vi "ep_Torque to Load.vi"(0 "air-gap torque waveform [Nm]":waveform(dbl), 1 "total input active power [W]":dbl, 5 "speed [RPM]":dbl, 11 "error in (no error)":errorcluster, 12 "initial conditions":T1) -> (3 "torque waveform [Nm]":waveform(dbl), 4 "torque [Nm]":dbl, 6 "load [W]":dbl, 8 "efficiency [%]":dbl, 14 "final conditions":T1, 15 "error out":errorcluster)   [LabVIEW 2014, in "NI_EP_Motor Monitoring.lvlib"]
uses:
  <vilib>/addons/Electrical Power/Motor Monitoring/NI_EP_Motor Monitoring.lvlib
  <vilib>/addons/Electrical Power/Motor Monitoring/subVIs/ep_Initial Conditions for Air Gap.ctl
  <vilib>/Analysis/baseanly.llb/Mean (DBL).vi
  <vilib>/Analysis/NI_AALBase.lvlib
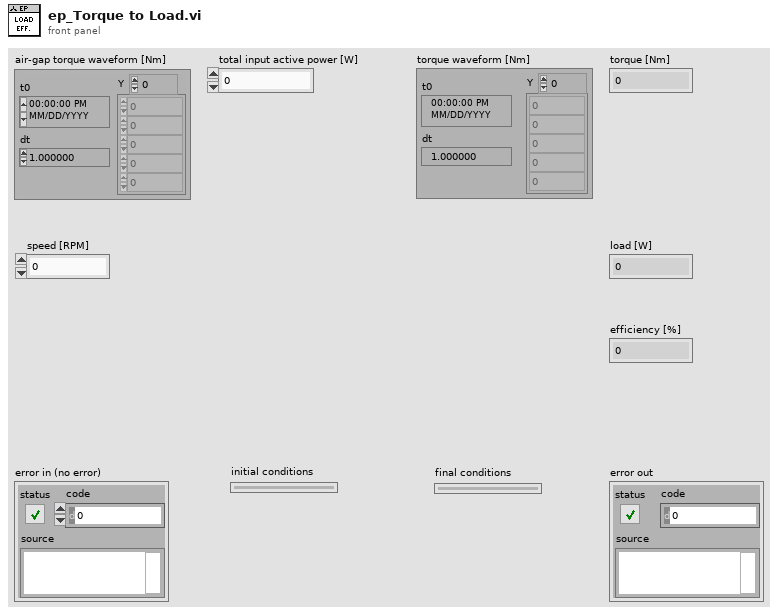
[diagram p1: front panel]
types:
  T1 = typedef "NI_EP_Motor Monitoring.lvlib/ep_Initial Conditions for Air Gap.ctl" = cluster{"integration state in A":cluster{"initial value":dbl, "initial integration":dbl}, "integration state in B":cluster{"initial value":dbl, "initial integration":dbl}, "integrated state A":dbl[], "integrated state B":dbl[], "previous length":i32, "loss and polepair":cluster{"Pstray [W]":dbl, "Pfric [W]":dbl, "Polepair #":i32, "synchronous speed [RPM]":dbl}, "expected timestamp":timestamp}
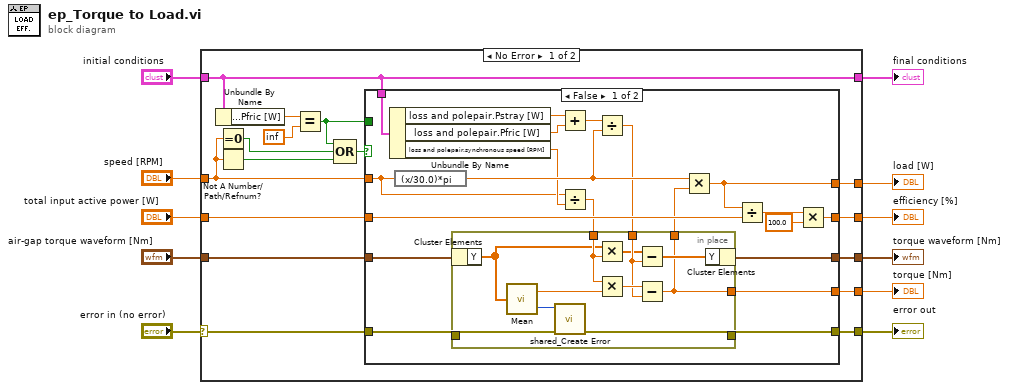
[diagram p0: block diagram]
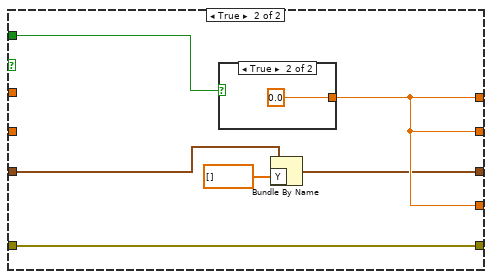
[diagram p2: hidden frame]
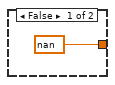
[diagram p3: hidden frame]
diagram:
  n1 = case shown="No Error" "error in (no error)" {
    selector: "error in (no error)" -> [w23 w67]
    tunnel: "initial conditions" -> [w15 _]
    tunnel: [w15 _] -> w1
    tunnel: [w22 w67] -> w10
    tunnel: "air-gap torque waveform [Nm]" -> [w27 _]
    tunnel: [w21 _] -> w8
    tunnel: "speed [RPM]" -> [w16 _]
    tunnel: [w26 _] -> w6
    tunnel: "total input active power [W]" -> [w25 _]
    tunnel: [w24 _] -> w4
    tunnel: [w20 _] -> w3
    frame No Error {
      n2 = Unbundle By Name(w15) -> ("loss and polepair.Pfric [W]"=w14:dbl)
      n3 = Equal To 0?(x=w16) -> (x = 0?=w17:bool)
      n4 = Not A Number/Path/Refnum?(number/path/refnum=w16) -> (NaN/Path/Refnum?=w18:bool)
      n5 = Equal?(x=w14, y=inf) -> (x = y?=w12:bool)
      n6 = Compound Arithmetic op=OR(w12, w17, w18) -> (w19:bool)
      n7 = case shown="False" w19 {
        tunnel: w27 -> [w30 w61]
        tunnel: w16 -> [w33 _]
        tunnel: [w47 w63] -> w26
        tunnel: w25 -> [w46 _]
        tunnel: [w43 w63] -> w24
        tunnel: w23 -> [w42 w64]
        tunnel: [w41 w64] -> w22
        tunnel: w15 -> [w40 _]
        tunnel: [w28 w63] -> w21
        tunnel: [w29 w62] -> w20
        tunnel: w12 -> [_ w59]
        frame False {
          n8 = Unbundle By Name(w40) -> ("loss and polepair.Pstray [W]"=w39:dbl, "loss and polepair.Pfric [W]"=w38:dbl, "loss and polepair.synchronous speed [RPM]"=w34:dbl)
          n9 = expression code="(x/30.0)*pi" ("RPM to radian/s")(w33) -> (w36:dbl)
          n10 = Add(x=w39, y=w38) -> (x+y=w37:dbl)
          n11 = Divide(x=w33, y=w34) -> (x/y=w31:dbl)
          n12 = Divide(x=w37, y=w36) -> (x/y=w32:dbl)
          n13 = in-place {
            in-place-border: w42 -> [w57]
            in-place-border: [w56] -> w41
            in-place-border: [w48] -> w35
            in-place-border: w32 -> [w53]
            in-place-border: w31 -> [w51]
            in-place-border: [w48] -> w28
            n14 = in-place-cluster #1(w30) -> ("Y"=w50:dbl[])
            n15 = call-poly <vilib>:"Mean.vi"("X"=w50) -> ("mean"=w55:dbl, "error"=w58:i32)
            n16 = call <vilib>:"shared_Create Error.vi"("error in (no error)"=w57, "error code (0)"=w58) -> ("error out"=w56:errorcluster)  [unwired: 9 in]
            n17 = Multiply(x=w50, y=w51) -> (x*y=w52:dbl[])
            n18 = Multiply(x=w51, y=w55) -> (x*y=w54:dbl)
            n19 = Subtract(x=w52, y=w53) -> (x-y=w49:dbl[])
            n20 = Subtract(x=w54, y=w53) -> (x-y=w48:dbl)
            n21 = in-place-cluster #1("Y"=w49) -> (w29:waveform(dbl))
          }
          n22 = Multiply(x=w36, y=w35) -> (x*y=w47:dbl)
          n23 = Divide(x=w47, y=w46) -> (x/y=w45:dbl)
          n24 = Multiply(x=w45, y=100.0) -> (x*y=w43:dbl)
        }
        frame True {
          n25 = case shown="True" w59 {
            tunnel: [nan 0.0] -> w63
            frame False {
            }
            frame True {
            }
          }
          n26 = Bundle By Name(cluster=w61, "Y"=dbl[] []) -> (w62:waveform(dbl))
        }
      }
    }
    frame Error {
    }
  }
  "error out" <- w10
  "torque [Nm]" <- w8
  "load [W]" <- w6
  "efficiency [%]" <- w4
  "torque waveform [Nm]" <- w3
  "final conditions" <- w1
